vi "getBounds.vi"(0 "reference":refnum<class "Graph.lvclass">, 1 "graphics":refnum<class "Graphics.lvclass">, 5 "error in (no error)":errorcluster) -> (14 "reference out":refnum<class "Graph.lvclass">, 15 "bounds":T1 {"height" format="%.2f"; "width" format="%.2f"; "y" format="%.2f"; "x" format="%.2f"}, 19 "error out":errorcluster)   [LabVIEW 2014, in "Graph.lvclass"]
doc: "public Rectangle2D getBounds(Graphics2D g2)"
uses:
  <resource>/Framework/Providers/Open_GDS/UML/Graph_class/Graph.lvclass
  <resource>/Framework/Providers/Open_GDS/UML/Graphics_class/Graphics.lvclass
  <resource>/Framework/Providers/Open_GDS/UML/General/Rectangle/Rectangle Rectangle2D.ctl
  <resource>/Framework/Providers/Open_GDS/UML/AbstractNode_class/AbstractNode.lvclass
  <resource>/Framework/Providers/Open_GDS/UML/AbstractEdge_class/AbstractEdge.lvclass
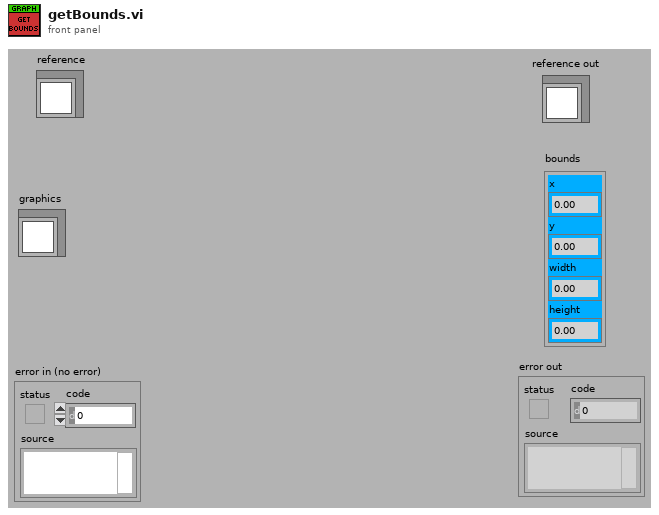
[diagram p1: front panel]
types:
  T1 = typedef "Rectangle Rectangle2D.ctl" = cluster{"x":dbl, "y":dbl, "width":dbl, "height":dbl}
  T2 = typedef "Graph.lvclass/ObjectAttributes.ctl" = cluster{"nodes":refnum<class "AbstractNode.lvclass">[], "edges":refnum<class "AbstractEdge.lvclass">[], "nodesToBeRemoved":refnum<class "AbstractNode.lvclass">[], "edgesToBeRemoved":refnum<class "AbstractEdge.lvclass">[], "needsLayout":bool, "LayoutNodes":refnum<class "AbstractNode.lvclass">[]}
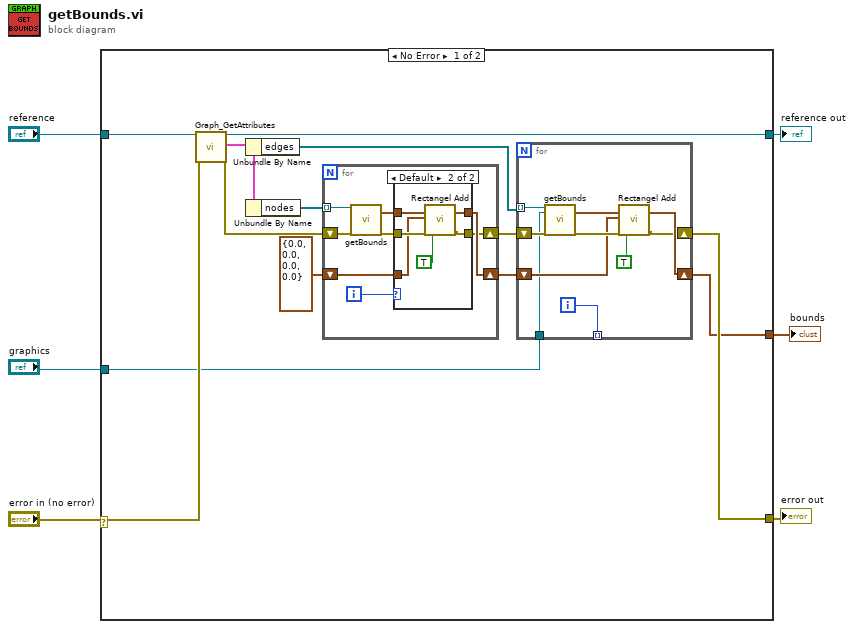
[diagram p0: block diagram]
diagram:
  n1 = case shown="No Error" "error in (no error)" {
    selector: "error in (no error)" -> [w16 w46]
    tunnel: "reference" -> [w19 w47]
    tunnel: [w18 w46] -> w5
    tunnel: [w17 w47] -> w4
    tunnel: "graphics" -> [w15 _]
    tunnel: [w14 _] -> w1
    frame No Error {
      n2 = call <resource>:"Graph_GetAttributes.vi"("reference in"=w19, "error in (no error)"=w16) -> ("reference out"=w17:refnum<class "Graph.lvclass">, "Data"=w7:T2, "error out"=w8:errorcluster)  [unwired: 1 in, 14 out]
      n3 = Unbundle By Name(w7) -> ("edges"=w9:refnum<class "AbstractEdge.lvclass">[])
      n4 = Unbundle By Name(w7) -> ("nodes"=w13:refnum<class "AbstractNode.lvclass">[])
      n5 = for {
        shift-right: [w31] -> w10
        shift-left: w8 -> [w37]
        tunnel: w13 -> [w36] mode=indexing
        shift-right: [w32] -> w11
        shift-left: T1 {"x"=0.0, "y"=0.0, "width"=0.0, "height"=0.0} ("boundsAdded") -> [w33]
        i -> [w30]
        n6 = call-dynamic "getBounds.vi"("reference"=w36, "error in (no error)"=w37) -> ("bounds"=w35:T1, "error out"=w34:errorcluster)  [unwired: 15 in, 1 out]
        n7 = case shown="Default" w30 {
          tunnel: w35 -> [w39 w45]
          tunnel: w34 -> [w38 w44]
          tunnel: w33 -> [_ w43]
          tunnel: [w39 w42] -> w32
          tunnel: [w38 w41] -> w31
          frame 0 {
          }
          frame Default {
            n8 = call <resource>:"Rectangel Add.vi"("bounds1"=w45, "bounds2"=w43, "error in (no error)"=w44, "useAbsoluteCordinates(False)"=TRUE) -> ("boundsAdded"=w42:T1, "error out"=w41:errorcluster)  [unwired: 1 in, 13 out]
          }
        }
      }
      n9 = for {
        shift-right: [w23] -> w18
        shift-left: w10 -> [w29]
        tunnel: w9 -> [w28] mode=indexing
        shift-right: [w24] -> w14
        shift-left: w11 -> [w25]
        tunnel: w15 -> [w22]
        tunnel: [w20] -> _ mode=indexing
        i -> [w20]
        n10 = call-dynamic "getBounds.vi"("reference"=w28, "graphics"=w22, "error in (no error)"=w29) -> ("bounds"=w27:T1, "error out"=w26:errorcluster)  [unwired: 14 in, 1 out]
        n11 = call <resource>:"Rectangel Add.vi"("bounds1"=w27, "bounds2"=w25, "error in (no error)"=w26, "useAbsoluteCordinates(False)"=TRUE) -> ("boundsAdded"=w24:T1, "error out"=w23:errorcluster)  [unwired: 1 in, 13 out]
      }
    }
    frame Error {
    }
  }
  "reference out" <- w4
  "error out" <- w5
  "bounds" <- w1
